vi "Threshold_Detection.vi"(1 "Threshold Value":dbl, 2 "Length of Array":i32, 3 "Array":dbl[](array[numeric])) -> (0 "Detection Index":i32)   [LabVIEW 2023]
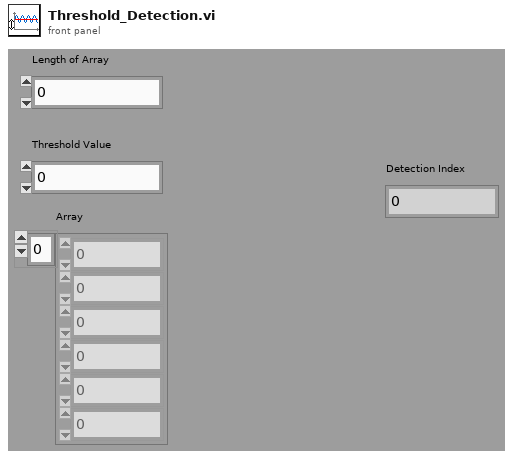
[diagram p1: front panel]
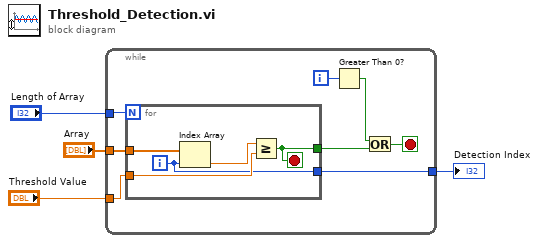
[diagram p0: block diagram]
diagram:
  n1 = while {
    tunnel: "Array" -> [w12]
    tunnel: "Threshold Value" -> [w11]
    tunnel: [w10] -> w2
    tunnel: "Length of Array" -> [w9]
    i -> [w8]
    stop <- w7 stop-if-true
    n2 = for {
      N: w9 -> [_]
      tunnel: w12 -> [w17]
      tunnel: w11 -> [w15]
      tunnel: [w13] -> w5
      tunnel: [w14] -> w10
      i -> [w14]
      stop <- w13 stop-if-true
      n3 = Index Array "Index Array"(array=w17, index=w14) -> (element=w16:dbl)
      n4 = Greater Or Equal?(x=w16, y=w15) -> (x >= y?=w13:bool)
    }
    n5 = Greater Than 0?(x=w8) -> (x > 0?=w6:bool)
    n6 = Or(x=w6, y=w5) -> (x .or. y?=w7:bool)
  }
  "Detection Index" <- w2
